vi "inst.vi"(11 "Platter in":T1 format="%032b") -> (3 "instruction":T1 format="%032b")   [LabVIEW 2020]
uses:
  Platter.ctl
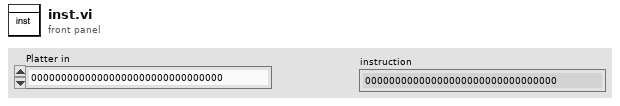
[diagram p1: front panel]
types:
  T1 = typedef "Platter.ctl" = u32
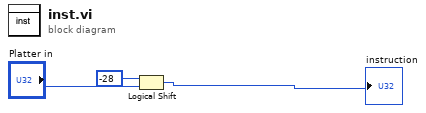
[diagram p0: block diagram]
diagram:
  n1 = Logical Shift(y=i16 -28, x="Platter in") -> (x << y=→"instruction":T1)
